vi "Destroy.vi"(8 "error in (no error)":errorcluster, 11 "obj":refnum<class "SciWare_ByRefActiveObj_V1.0.0.lvclass">) -> (0 "error out":errorcluster)   [LabVIEW 2009, in "SciWare_ByRefActiveObj_V1.0.0.lvclass"]
doc: "Destroys the by ref object.\n\nBSD License (http://www.opensource.org/licenses/bsd-license.php)"
uses:
  SciWare_ByRefActiveObj_V1.0.0.lvclass
  SciWare_ByRefActiveObj_V1.0.0.lvclass/SciWare_ByRefActiveObj_V1.0.0.ctl
panel:
  # "BSD License (http://www.opensource.org/licenses/bsd-license.php)"
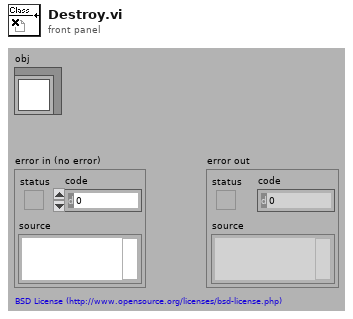
[diagram p1: front panel]
types:
  T1 = typedef "SciWare_ByRefActiveObj_V1.0.0.lvclass/DataRef.ctl" = refnum<data-value>
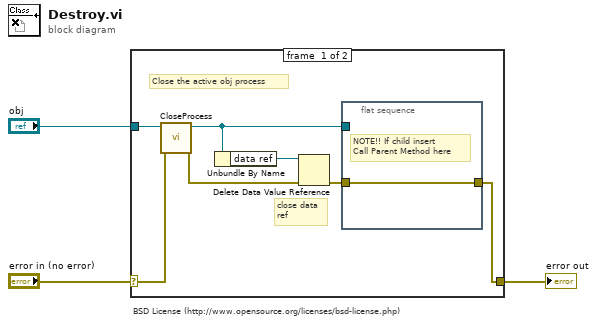
[diagram p0: block diagram]
diagram:
  # "BSD License (http://www.opensource.org/licenses/bsd-license.php)"
  n1 = case shown="No Error" "error in (no error)" {
    selector: "error in (no error)" -> [w8 w12]
    tunnel: [w5 w12] -> w2
    tunnel: "obj" -> [w9 _]
    frame #0 {
      # "close data\nref"
      # "Close the active obj process"
      n2 = call-dynamic "CloseProcess.vi"("error in (no error)"=w8, "obj"=w9) -> ("error out"=w7:errorcluster, "obj out"=w4:refnum<class "SciWare_ByRefActiveObj_V1.0.0.lvclass">)  [unwired: 8 in]
      n3 = Unbundle By Name(w4) -> ("data ref"=w10:T1)
      n4 = Delete Data Value Reference(data value reference=w10, error in=w7) -> (error out=w6:errorcluster)  [unwired: 1 out]
      n5 = flat-sequence {
        tunnel: w6 -> [w11]
        tunnel: [w11] -> w5
        tunnel: w4 -> [_]
        frame #0 {
          # "NOTE!! If child insert\nCall Parent Method here"
        }
      }
    }
    frame #1 {
    }
  }
  "error out" <- w2
